vi "上传到MDSplus.vi"(5 "Channel":string[](array[string]), 6 "上传参数":cluster{"tree name":string, "host IP":string}, 7 "Group":string, 8 "error in (no error)":errorcluster, 9 "Time":sgl, 10 "Rate":sgl, 11 "file path":path) -> (0 "error out":errorcluster, 3 "State":string)   [LabVIEW 2018]
uses:
  Mdsplus/MDSplusVBC.dll
panel:
  in  "shot number":i32
  in  "数组":sgl[](array[numeric])
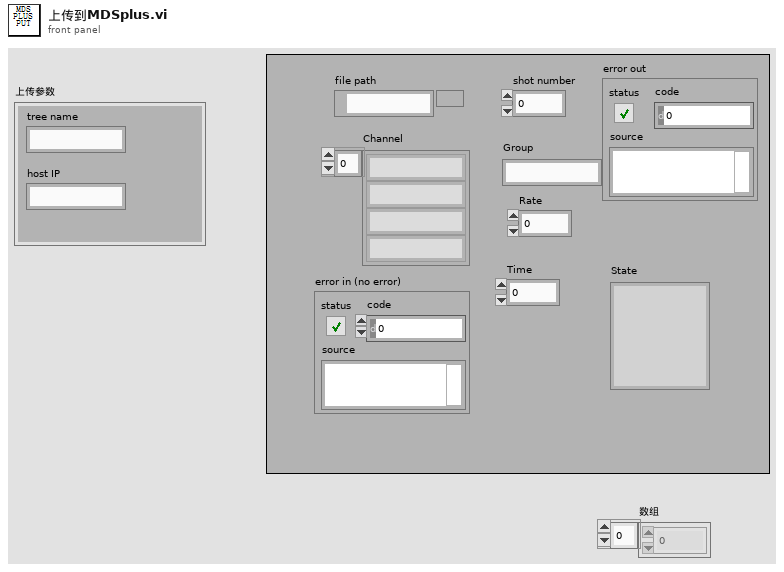
[diagram p1: front panel]
types:
  T1 = enum16{"open", "open or create", "create or replace", "create", "open (read-only)"}
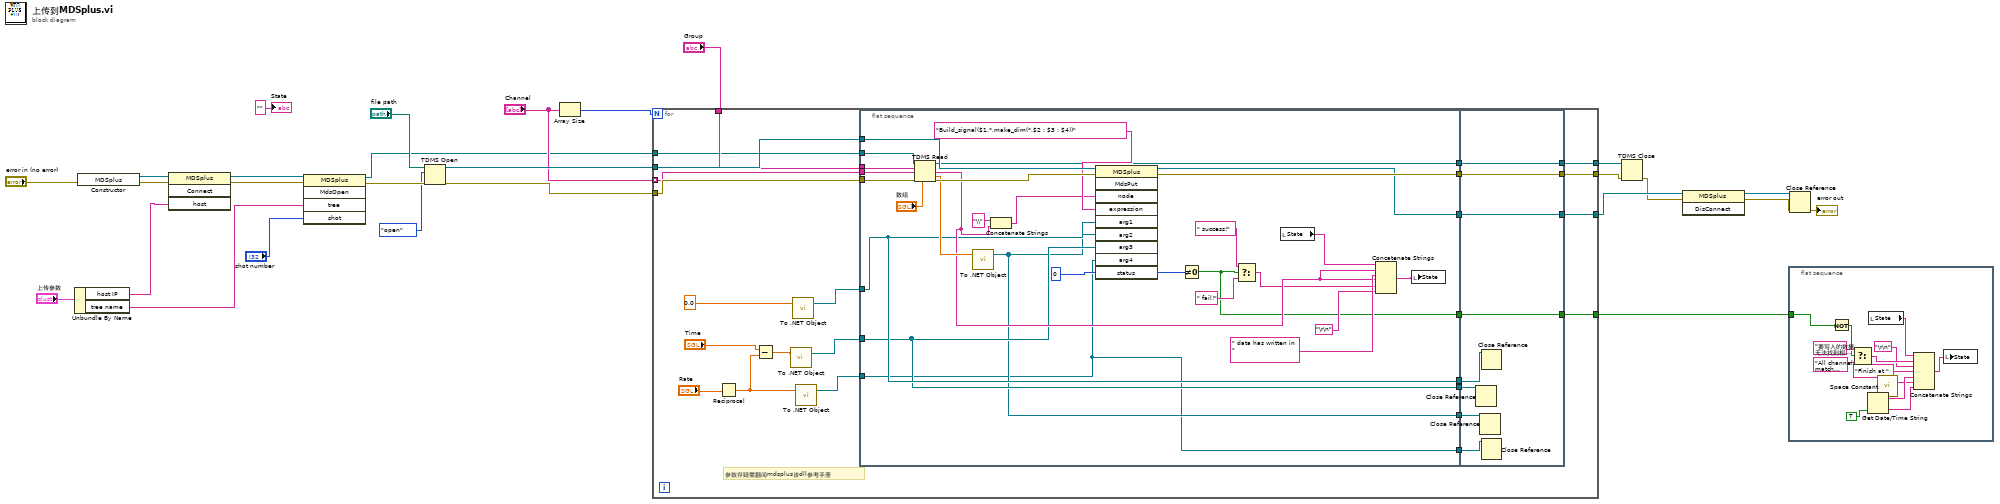
[diagram p0: block diagram]
diagram:
  n1 = Unbundle By Name("上传参数") -> ("host IP"=w2:string, "tree name"=w1:string)
  n2 = constructor class="MDSplus"(error in="error in (no error)") -> (reference out=w26:refnum<k24>, error out=w25:errorcluster)  [unwired: 2 in, 1 out]
  n3 = invoke class="MDSplus" method="Connect"(reference=w26, error in=w25, "host"=w2) -> (reference out=w24:refnum<k24>, error out=w23:errorcluster)  [unwired: 1 in, 2 out]
  n4 = invoke class="MDSplus" method="MdsOpen"(reference=w24, error in=w23, "tree"=w1, "shot"="shot number") -> (reference out=w12:refnum<k24>, error out=w20:errorcluster)  [unwired: 1 in, 3 out]
  n5 = TDMS Open(8:w20, 10:T1."open" ("operation (0:open)"), 11:"file path") -> (0:w15:errorcluster, 3:w16:refnum<k34>)  [unwired: 4 in]
  n6 = Array Size(array="Channel") -> (size(s)=w17:i32)
  n7 = for {
    N: w17 -> [_]
    tunnel: w16 -> [w47]
    tunnel: w15 -> [w46]
    tunnel: "Group" -> [w45]
    tunnel: "Channel" -> [w44] mode=indexing
    tunnel: w12 -> [w43]
    tunnel: [w35] -> w11
    tunnel: [w33] -> w10
    tunnel: [w31] -> w9
    tunnel: [w28] -> w4
    # "参数存疑需翻阅mdsplus该dll参考手册"
    n8 = Reciprocal(x="Rate") -> (1/x=w49:sgl)
    n9 = Subtract(x="Time", y=w49) -> (x-y=w48:sgl)
    n10 = call <vilib>:"To .NET Object.vi"("anything"=w48) -> (".NET object"=w41:refnum<k24>)  [unwired: 1 in, 1 out]
    n11 = call <vilib>:"To .NET Object.vi"("anything"=sgl 0.0) -> (".NET object"=w42:refnum<k24>)  [unwired: 1 in, 1 out]
    n12 = call <vilib>:"To .NET Object.vi"("anything"=w49) -> (".NET object"=w40:refnum<k24>)  [unwired: 1 in, 1 out]
    n13 = flat-sequence {
      tunnel: w47 -> [w81]
      tunnel: w46 -> [w80]
      tunnel: w45 -> [w79]
      tunnel: w44 -> [w78]
      tunnel: w43 -> [w75]
      tunnel: w42 -> [w60]
      tunnel: w41 -> [w59]
      tunnel: w40 -> [w57]
      tunnel: [w60] -> w39
      tunnel: [w59] -> w38
      tunnel: [w58] -> w37
      tunnel: [w57] -> w36
      tunnel: [w56] -> w34
      tunnel: [w55] -> w32
      tunnel: [w54] -> w30
      tunnel: [w53] -> w29
      tunnel: w39 -> [w89]
      tunnel: w38 -> [w88]
      tunnel: w37 -> [w87]
      tunnel: w36 -> [w86]
      tunnel: [w85] -> w35
      tunnel: w34 -> [w85]
      tunnel: [w84] -> w33
      tunnel: w32 -> [w84]
      tunnel: [w83] -> w31
      tunnel: w30 -> [w83]
      tunnel: w29 -> [w82]
      tunnel: [w82] -> w28
      frame #0 {
        n14 = TDMS Read(0:w81, 5:w79, 7:w78, 11:w80, 12:"数组") -> (4:w56:refnum<k34>, 8:w64:string, 10:w71:sgl[], 15:w76:errorcluster)  [unwired: 3 in, 2 out]
        n15 = call <vilib>:"To .NET Object.vi"("anything"=w71) -> (".NET object"=w58:refnum<k24>)  [unwired: 1 in, 1 out]
        n16 = Concatenate Strings("\\" ("string"), w64) -> (w72:string)
        n17 = invoke class="MDSplus" method="MdsPut"(reference=w75, error in=w76, "node"=w72, "expression"="Build_signal($1,*,make_dim(*,$2 : $3 : $4))", "arg1"=w58, "arg2"=w60, "arg3"=w59, "arg4"=w57, "status"=0) -> (reference out=w54:refnum<k24>, error out=w55:errorcluster, "status"=w69:i32)  [unwired: 1 in, 7 out]
        n18 = Not Equal To 0?(x=w69) -> (x != 0?=w53:bool)
        n19 = Select(t=" success!", s=w53, f=" fail!") -> (s? t:f=w63:string)
        n20 = local read "State"() -> (w66:string)
        n21 = Concatenate Strings(w66, w64, " data has written in ", w64, w63, "\r\n") -> (w61:string)
        n22 = local write "State"(w61) -> ()
      }
      frame #1 {
        n23 = Close Reference(reference=w88) -> ()  [unwired: 1 in, 1 out]
        n24 = Close Reference(reference=w87) -> ()  [unwired: 1 in, 1 out]
        n25 = Close Reference(reference=w89) -> ()  [unwired: 1 in, 1 out]
        n26 = Close Reference(reference=w86) -> ()  [unwired: 1 in, 1 out]
      }
    }
  }
  n27 = TDMS Close(8:w10, 11:w11) -> (0:w8:errorcluster)  [unwired: 1 out]
  n28 = invoke class="MDSplus" method="DisConnect"(reference=w9, error in=w8) -> (reference out=w7:refnum<k24>, error out=w6:errorcluster)  [unwired: 1 in, 1 out]
  n29 = flat-sequence {
    tunnel: w4 -> [w91]
    frame #0 {
      n30 = Not(x=w91) -> (.not. x?=w90:bool)
      n31 = Select(t="要写入的数据无法找到相应的通道！", s=w90, f="All channels match success.") -> (s? t:f=w100:string)
      n32 = Get Date/Time String(want seconds? (F)=TRUE ("需要秒？(F)")) -> (date string=w94:string, time string=w93:string)  [unwired: 2 in]
      n33 = local read "State"() -> (w101:string)
      n34 = call <vilib>:"Space Constant.vi"() -> ("String"=w92:string)
      n35 = Concatenate Strings(w101, w100, "\r\n", "Finish at " ("字符串"), w94, w92, w93) -> (w102:string)
      n36 = local write "State"(w102) -> ()
    }
  }
  n37 = Close Reference(reference=w7, error in (no error)=w6) -> (error out=→"error out":errorcluster)
  "State" <- "" ("State")
